vi "Test Vector from File.vi"(8 "error in (no error)":errorcluster, 11 "Test Vector Demo In":refnum<class "Test Vector Demo.lvclass">) -> (0 "error out":errorcluster, 3 "Test Vector Demo Out":refnum<class "Test Vector Demo.lvclass">)   [LabVIEW 2020, in "Test Vector Demo.lvclass"]
uses:
  Test Vector Demo.lvclass
  C:/Users/anton/Documents/GitHub/LUnit/source/Framework/Test Vector/LUnit Test Vector.lvclass
  Framework/Test Vector/LUnit Test Vector.lvclass
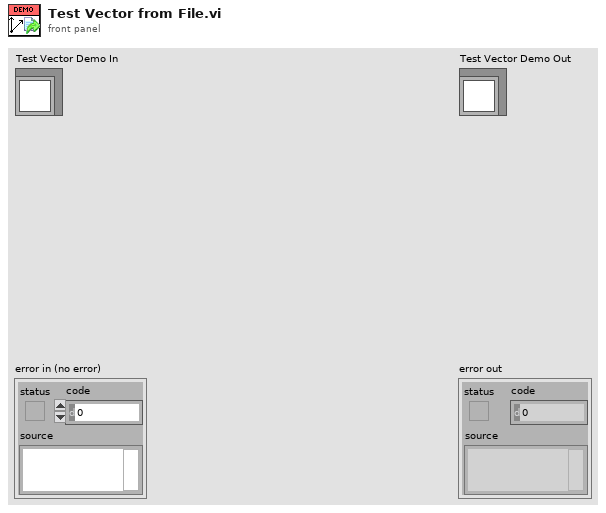
[diagram p1: front panel]
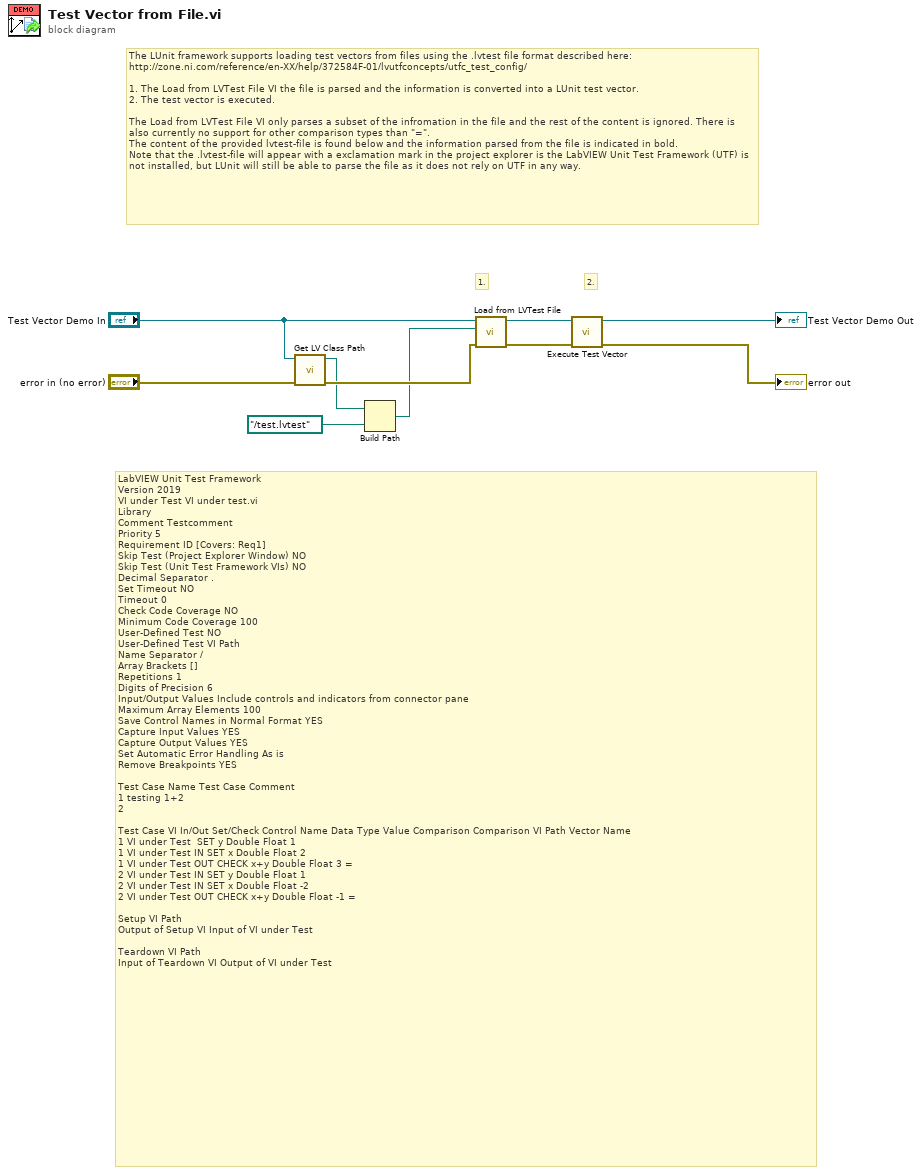
[diagram p0: block diagram]
diagram:
  # "2."
  # "1."
  # "The LUnit framework supports loading test vectors from files using the .lvtest file format described here:\nhttp://zone.ni.com/reference/en-XX/help/372584F-01/lvutfconcepts/utfc_test_config/\n \n1. The Load from LVTest File VI the file is parsed and the information is converted into a LUnit test vector. \n2. The test vector is executed.\n\nThe Load from LVTest File VI only parses a subset of the infromation in the file and the rest of the content is ignored. There is also currently no support for other comparison types than \"=\".\nThe content of the provided lvtest-file is found below and the information parsed from the file is indicated in bold.\nNote that the .lvtest-file will appear with a exclamation mark in the project explorer is the LabVIEW Unit Test Framework (UTF) is not installed, but LUnit will still be able to parse the file as it does not rely on UTF in any way."
  # "LabVIEW Unit Test Framework\t \nVersion\t2019\nVI under Test\tVI under test.vi\nLibrary\t\nComment\tTestcomment\nPriority\t5\nRequirement ID\t[Covers: Req1]\nSkip Test (Project Explorer Window)\tNO\nSkip Test (Unit Test Framework VIs)\tNO\nDecimal Separator\t.\nSet Timeout\tNO\nTimeout\t0\nCheck Code Coverage\tNO\nMinimum Code Coverage\t100\nUser-Defined Test\tNO\nUser-Defined Test VI Path\t\nName Separator\t/\nArray Brackets\t[]\nRepetitions\t1\nDigits of Precision\t6\nInput/Output Values\tInclude controls and indicators from connector pane\nMaximum Array Elements\t100\nSave Control Names in Normal Format\tYES\nCapture Input Values\tYES\nCapture Output Values\tYES\nSet Automatic Error Handling\tAs is\nRemove Breakpoints\tYES\n\nTest Case Name\tTest Case Comment\n1\ttesting 1+2\n2\t\n\nTest Case\tVI\tIn/Out\tSet/Check\tControl Name\tData Type\tValue\tComparison\tComparison VI Path\tVector Name\n1\tVI under Test\t\tSET\ty\tDouble Float\t1\t\t\t\n1\tVI under Test\tIN\tSET\tx\tDouble Float\t2\t\t\t\n1\tVI under Test\tOUT\tCHECK\tx+y\tDouble Float\t3\t=\t\t\n2\tVI under Test\tIN\tSET\ty\tDouble Float\t1\t\t\t\n2\tVI under Test\tIN\tSET\tx\tDouble Float\t-2\t\t\t\n2\tVI under Test\tOUT\tCHECK\tx+y\tDouble Float\t-1\t=\t\t\n\nSetup VI Path\t\nOutput of Setup VI\tInput of VI under Test\n\nTeardown VI Path\t\nInput of Teardown VI\tOutput of VI under Test"
  n1 = call <vilib>:"Get LV Class Path.vi"("error in (no error)"="error in (no error)", "object"="Test Vector Demo In") -> ("error out"=w10:errorcluster, "class path"=w7:path)  [unwired: 8 in]
  n2 = Build Path(base path=w7, name or relative path=path "../test.lvtest" ("VI Under Test Path")) -> (appended path=w6:path)
  n3 = call "Load from LVTest File.vi"("error in (no error)"=w10, "LVTest File Path"=w6, "LUnit Test Vector In"="Test Vector Demo In") -> ("error out"=w5:errorcluster, "LUnit Test Vector Out"=w4:refnum<class "Test Vector Demo.lvclass">)  [unwired: 7 in]
  n4 = call "Execute Test Vector.vi"("error in (no error)"=w5, "LUnit Test Vector in"=w4) -> ("error out"=→"error out":errorcluster, "LUnit Test Vector out"=→"Test Vector Demo Out":refnum<class "Test Vector Demo.lvclass">)  [unwired: 8 in]
